vi "Write PCM channel.vi"(8 "error in (no error)":errorcluster, 10 "PCM channel":u8, 11 "Solenoids in":refnum<class "Solenoids.lvclass">) -> (0 "error out":errorcluster, 3 "Solenoids out":refnum<class "Solenoids.lvclass">)   [LabVIEW 2019, in "Pneumatics control.lvlib" / "Solenoids.lvclass"]
uses:
  Solenoids.lvclass
  Solenoids.lvclass/Solenoids.ctl
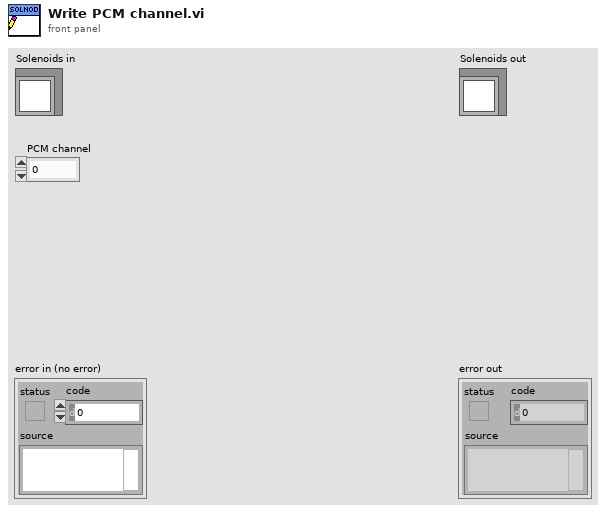
[diagram p1: front panel]
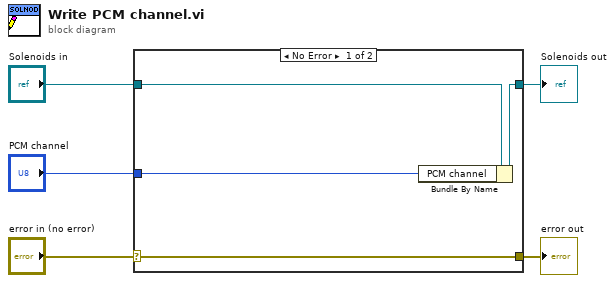
[diagram p0: block diagram]
diagram:
  n1 = case shown="No Error" "error in (no error)" {
    selector: "error in (no error)" -> [w9 w10]
    tunnel: [w9 w10] -> w4
    tunnel: [w7 w11] -> w2
    tunnel: "Solenoids in" -> [w8 w11]
    tunnel: "PCM channel" -> [w6 _]
    frame No Error {
      n2 = Bundle By Name(cluster=w8, "PCM channel"=w6) -> (w7:refnum<class "Solenoids.lvclass">)
    }
    frame Error {
    }
  }
  "error out" <- w4
  "Solenoids out" <- w2
